vi "PID Controller.vi"(6 "dt":dbl=1.0 format="%0.2f", 7 "Initialize":bool, 8 "Previous Set Point":dbl format="%0.2f", 9 "Desired Setpoint":dbl format="%0.2f", 10 "Measured":dbl format="%0.2f", 11 "PID Parameters":T1) -> (0 "New Setpoint":dbl, 2 "Error":dbl)   [LabVIEW 2010]
uses:
  <vilib>/ptbypt/NI_PtbyPt.lvlib
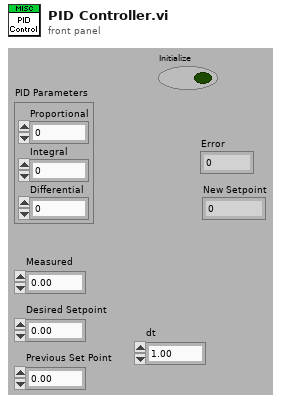
[diagram p1: front panel]
types:
  T1 = cluster{"Proportional":dbl, "Integral":dbl, "Differential":dbl}
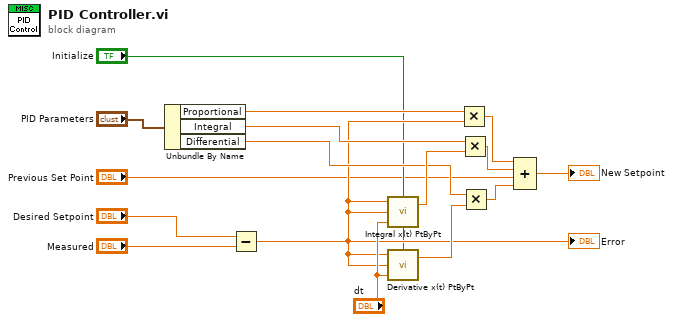
[diagram p0: block diagram]
diagram:
  n1 = Unbundle By Name("PID Parameters") -> ("Proportional"=w10:dbl, "Integral"=w9:dbl, "Differential"=w7:dbl)
  n2 = Subtract(x="Desired Setpoint", y="Measured") -> (x-y=w4:dbl)
  "Error" <- w4
  n3 = call <vilib>:"Integral x(t) PtByPt.vi"("initialize"="Initialize", "dt"="dt", "initial condition"=w4, "x"=w4) -> ("integral x(t)"=w16:dbl)  [unwired: 1 out]
  n4 = call <vilib>:"Derivative x(t) PtByPt.vi"("initialize"="Initialize", "dt"="dt", "initial condition"=w4, "x"=w4) -> ("dx/dt"=w6:dbl)  [unwired: 1 out]
  n5 = Multiply(x=w10, y=w4) -> (x*y=w13:dbl)
  n6 = Multiply(x=w9, y=w16) -> (x*y=w14:dbl)
  n7 = Multiply(x=w7, y=w6) -> (x*y=w5:dbl)
  n8 = Compound Arithmetic op=ADD(w13, w14, "Previous Set Point", w5) -> (→"New Setpoint":dbl)
